vi "Com_Matrix220_Connection Check.vi"(8 "error in":errorcluster, 11 "Buffer Data In":T1) -> (0 "error out":errorcluster, 2 "Timeout?":bool, 3 "Buffer Data Out":T1)   [LabVIEW 2016]
uses:
  Data Def/Com_Matrix220_Buffer Data.ctl
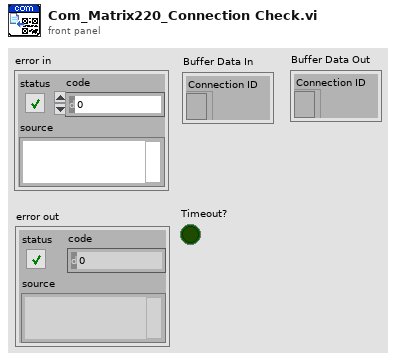
[diagram p1: front panel]
types:
  T1 = typedef "Com_Matrix220_Buffer Data.ctl" = cluster{"Connection ID":refnum<k5>}
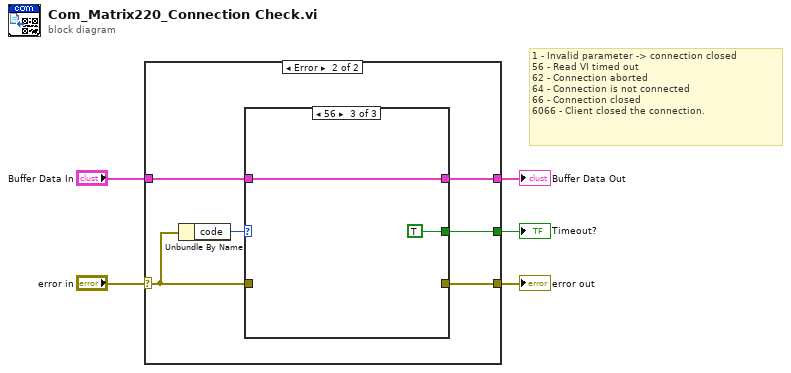
[diagram p0: block diagram]
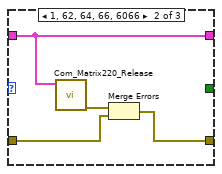
[diagram p4: hidden frame]
diagram:
  # "1 - Invalid parameter -> connection closed\n56 - Read VI timed out\n62 - Connection aborted\n64 - Connection is not connected\n66 - Connection closed\n6066 - Client closed the connection."
  n1 = case shown="Error" "error in" {
    selector: "error in" -> [w7 w12]
    tunnel: "Buffer Data In" -> [w6 w10]
    tunnel: [w7 w11] -> w3
    tunnel: [w6 w9] -> w2
    tunnel: [_ w8] -> w1
    frame No Error {
    }
    frame Error {
      n2 = Unbundle By Name(w12) -> ("code"=w13:i32)
      n3 = case shown="56" w13 {
        tunnel: w12 -> [w15 w18 _]
        tunnel: [w15 w17 _] -> w11
        tunnel: w10 -> [w14 w16 w21]
        tunnel: [w14 w16 w21] -> w9
        tunnel: [_ _ TRUE] -> w8
        frame Default {
        }
        frame 1, 62, 64, 66, 6066 {
          n4 = call "Com_Matrix220_Release.vi"("Buffer Data"=w16) -> ("error out"=w19:errorcluster)  [unwired: 10 in]
          n5 = Merge Errors(w19, w18) -> (w17:errorcluster)
        }
        frame 56 {
        }
      }
    }
  }
  "error out" <- w3
  "Buffer Data Out" <- w2
  "Timeout?" <- w1
